vi "Update.vi"(8 "error in":errorcluster, 10 "object ref in":T1, 11 "Multi Column Listbox in":refnum<class "Multi Column Listbox.lvclass">) -> (0 "error out":errorcluster, 2 "object ref out":T1, 3 "Multi Column Listbox out":refnum<class "Multi Column Listbox.lvclass">)   [LabVIEW 2013, in "Table Manager.lvlib" / "Multi Column Listbox.lvclass"]
uses:
  Multi Column Listbox.lvclass
  TagSelectModule/Source/editor node/object ref.ctl
  TagSelectModule/Source/editor node/tag select module editor node.lvclass
  <vilib>/NI/Tag Bus Data Framework/Configuration Editor/Classes/Engine Parent/Engine Parent Editor Node.lvclass
  Multi Column Listbox.lvclass/Multi Column Listbox.ctl
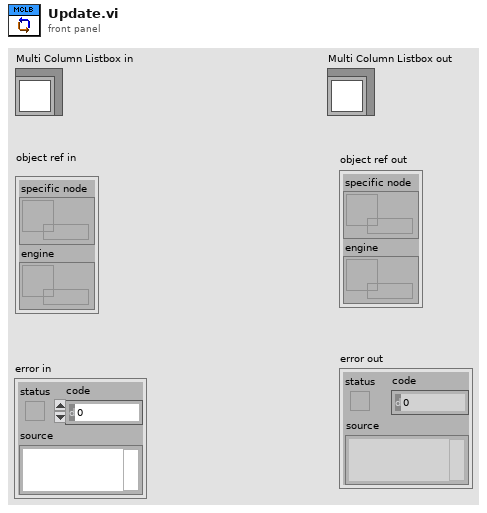
[diagram p1: front panel]
types:
  T1 = typedef "tag select module editor node.lvclass/object ref.ctl" = cluster{"specific node":refnum<data-value>, "engine":refnum<data-value>}
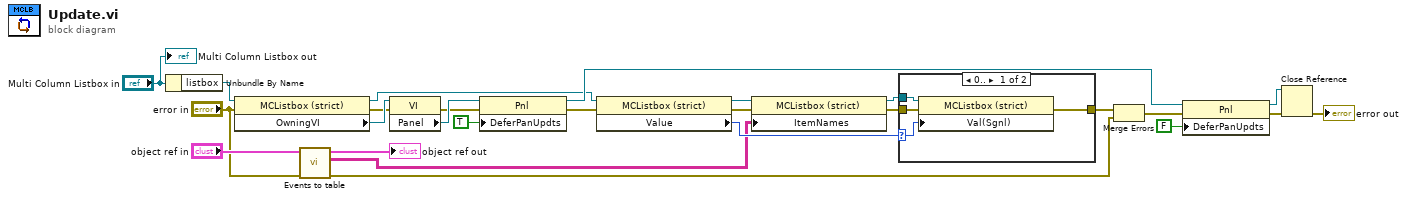
[diagram p0: block diagram]
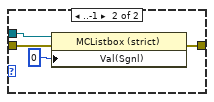
[diagram p2: hidden frame]
diagram:
  n1 = Unbundle By Name("Multi Column Listbox in") -> ("listbox"=w6:refnum<vi>)
  n2 = property class="MCListbox (strict)"(reference=w6, error in="error in") -> (reference out=w20:refnum<vi>, error out=w18:errorcluster, "OwningVI"=w19:refnum<vi>)
  n3 = call "Events to table.vi"("error in (no error)"="error in", "object ref in"="object ref in") -> ("error out"=w2:errorcluster, "table"=w8:string[][], "object ref out"=→"object ref out":T1)  [unwired: 7 in]
  n4 = property class="VI"(reference=w19, error in=w18) -> (error out=w24:errorcluster, "Panel"=w25:refnum<vi>)  [unwired: 1 out]
  n5 = property class="Pnl"(reference=w25, error in=w24, "DeferPanUpdts"=TRUE ("Defer Panel Updates")) -> (reference out=w22:refnum<vi>, error out=w11:errorcluster)
  n6 = property class="MCListbox (strict)"(reference=w20, error in=w11) -> (reference out=w16:refnum<vi>, error out=w12:errorcluster, "Value"=w13:i32)
  n7 = property class="MCListbox (strict)"(reference=w16, error in=w12, "ItemNames"=w8) -> (reference out=w15:refnum<vi>, error out=w14:errorcluster)
  n8 = case shown="0.." w13 {
    selector: w13 -> [w27 _]
    tunnel: w15 -> [w30 w34]
    tunnel: w14 -> [w29 w33]
    tunnel: [w28 w32] -> w3
    frame 0.. {
      n9 = property class="MCListbox (strict)"(reference=w30, error in=w29, "Val(Sgnl)"=w27) -> (error out=w28:errorcluster)  [unwired: 1 out]
    }
    frame ..-1 {
      n10 = property class="MCListbox (strict)"(reference=w34, error in=w33, "Val(Sgnl)"=0 ("Value (Signaling)")) -> (error out=w32:errorcluster)  [unwired: 1 out]
    }
  }
  n11 = Merge Errors(w3, w2) -> (w1:errorcluster)
  n12 = property class="Pnl"(reference=w22, error in=w1, "DeferPanUpdts"=FALSE ("Defer Panel Updates")) -> (reference out=w17:refnum<vi>, error out=w21:errorcluster)
  n13 = Close Reference(reference=w17, error in (no error)=w21) -> (error out=→"error out":errorcluster)
  "Multi Column Listbox out" <- "Multi Column Listbox in"
